vi "PicoScope5000aRunBlock.vi"(7 "Acquisition Settings":T1={"preTriggerSamples"=0, "postTriggerSamples"=1000, "timebase"=2} {"postTriggerSamples" format="%_6p"; "preTriggerSamples" format="%_6p"}, 8 "error in (no error)":errorcluster, 11 "handle in":i16) -> (0 "error out":errorcluster, 3 "handle out":i16, 4 "timeIndisposedMs":dbl, 6 "Total Requested Samples":u64)   [LabVIEW 2020]
doc: "Calls ps5000aRunBlock"
uses:
  Acquisition Settings.ctl
  ps5000a.dll
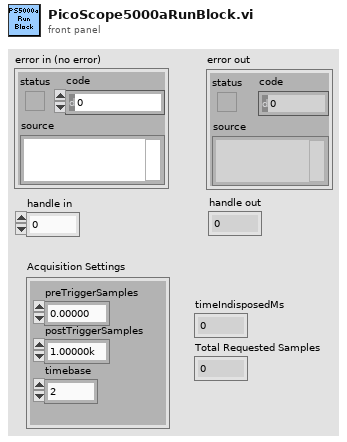
[diagram p1: front panel]
types:
  T1 = typedef "Acquisition Settings.ctl" = cluster{"preTriggerSamples":u64, "postTriggerSamples":u64, "timebase":u32}
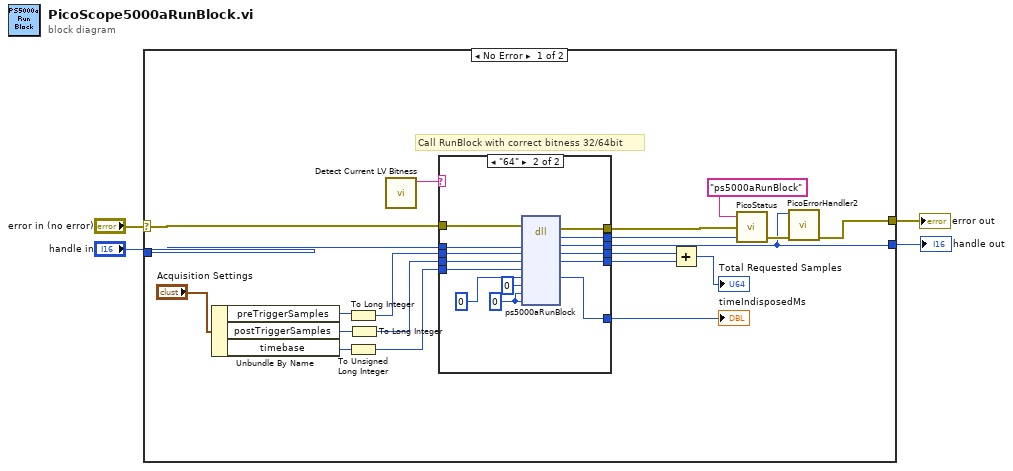
[diagram p0: block diagram]
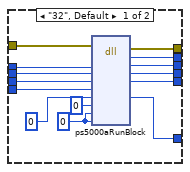
[diagram p2: hidden frame]
diagram:
  n1 = case shown="No Error" "error in (no error)" {
    selector: "error in (no error)" -> [w18 w54]
    tunnel: [w14 w54] -> w2
    tunnel: "handle in" -> [w17 w53]
    tunnel: [w13 w53] -> w3
    frame No Error {
      # "Call RunBlock with correct bitness 32/64bit"
      n2 = Unbundle By Name("Acquisition Settings") -> ("preTriggerSamples"=w10:u64, "postTriggerSamples"=w8:u64, "timebase"=w9:u32)
      n3 = To Long Integer(number=w10) -> (32bit integer=w7:i32)
      n4 = To Unsigned Long Integer(number=w9) -> (unsigned 32bit integer=w5:u32)
      n5 = To Long Integer(number=w8) -> (32bit integer=w6:i32)
      n6 = call "Detect Current LV Bitness.vi"() -> ("bitness"=w15:string)  [unwired: 11 in]
      n7 = case shown="\"64\"" w15 {
        tunnel: [w38 w52] -> w24
        tunnel: [w37 w51] -> w23
        tunnel: [w36 w50] -> w21
        tunnel: [w35 w49] -> w20
        tunnel: w18 -> [w34 w48]
        tunnel: w17 -> [w33 w47]
        tunnel: w7 -> [w31 w45]
        tunnel: w6 -> [w30 w44]
        tunnel: w5 -> [w29 w43]
        tunnel: [w28 w42] -> w13
        tunnel: [w25 w40] -> w12
        frame "32", Default {
          w27 = u32 0 ("pParameter")
          n8 = dll-call lib="ps5000a.dll" fn="ps5000aRunBlock" ("ps3000.dll:_ps3000_open_unit@0")(error in=w34, "handle"=w33, "noOfPreTriggerSamples"=w31, "noOfPostTriggerSamples"=w30, "timebase"=w29, "timeIndisposedMs"=0 ("pParameter"), "segmentIndex"=u32 0, "lpReady"=w27, "pParameter"=w27) -> (error out=w35:errorcluster, "PICO_STATUS"=w36:u32, "handle"=w28:i16, "noOfPreTriggerSamples"=w38:i32, "noOfPostTriggerSamples"=w37:i32, "timeIndisposedMs"=w25:i32)  [unwired: 6 in, 1 out]
        }
        frame "64" {
          w41 = u64 0 ("pParameter")
          n9 = dll-call lib="ps5000a.dll" fn="ps5000aRunBlock" ("ps3000.dll:_ps3000_open_unit@0")(error in=w48, "handle"=w47, "noOfPreTriggerSamples"=w45, "noOfPostTriggerSamples"=w44, "timebase"=w43, "timeIndisposedMs"=0 ("pParameter"), "segmentIndex"=u32 0, "lpReady"=w41, "pParameter"=w41) -> (error out=w49:errorcluster, "PICO_STATUS"=w50:u32, "handle"=w42:i16, "noOfPreTriggerSamples"=w52:i32, "noOfPostTriggerSamples"=w51:i32, "timeIndisposedMs"=w40:i32)  [unwired: 6 in, 1 out]
        }
      }
      "timeIndisposedMs" <- w12
      n10 = Add(x=w24, y=w23) -> (x+y=→"Total Requested Samples":i32)
      n11 = call "PicoStatus.vi"("PICO STATUS"=w21, "error in"=w20, "source"="ps5000aRunBlock") -> ("error out"=w16:errorcluster)
      n12 = call "PicoErrorHandler2.vi"("error in (no error)"=w16, "handle In"=w13) -> ("error out"=w14:errorcluster)  [unwired: 9 in]
    }
    frame Error {
    }
  }
  "error out" <- w2
  "handle out" <- w3
